vi "InterpolateData.vi"(7 "Interp. factor":i32=4, 8 "error in (no error)":errorcluster, 10 "Time":dbl[](array[numeric]), 11 "Array":cdb[][](array[numeric])) -> (0 "error out":errorcluster, 3 "Array interpolated":cdb[][](array[numeric]))   [LabVIEW 2017, in "AppPlugins.lvlib" / "ModelValidationPlugin.lvclass"]
uses:
  ModelValidationPlugin.lvclass
  <vilib>/gmath/NI_Gmath.lvlib
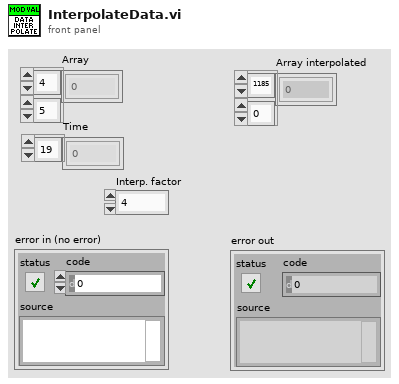
[diagram p1: front panel]
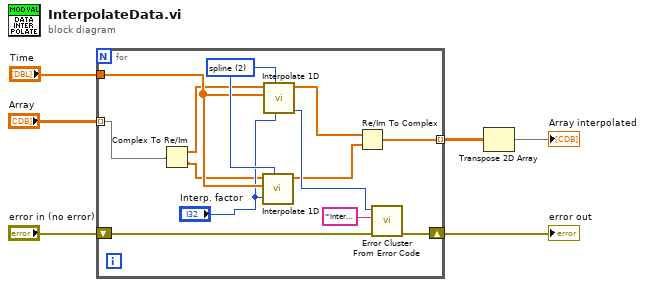
[diagram p0: block diagram]
diagram:
  n1 = for {
    shift-right: [w15] -> w5
    shift-left: "error in (no error)" -> [w16]
    tunnel: "Array" -> [w12] mode=indexing
    tunnel: "Time" -> [w18]
    tunnel: [w7] -> w3 mode=indexing
    w19 = 2 items=["nearest", "linear", "spline", "cubic Hermite", "Lagrange"] ("method")
    n2 = Complex To Re/Im(x + iy=w12) -> (x=w11:dbl[], y=w10:dbl[])
    n3 = call <vilib>:"Interpolate 1D.vi"("ntimes"="Interp. factor", "method"=w19, "X"=w18, "Y"=w10) -> ("yi"=w8:dbl[])  [unwired: 5 in, 2 out]
    n4 = call <vilib>:"Interpolate 1D.vi"("ntimes"="Interp. factor", "method"=w19, "X"=w18, "Y"=w11) -> ("error"=w17:i32, "yi"=w9:dbl[])  [unwired: 5 in, 1 out]
    n5 = Re/Im To Complex(1:w8, 2:w9) -> (0:w7:cdb[])
    n6 = call <vilib>:"Error Cluster From Error Code.vi"("error in (no error)"=w16, "error message (\"\")"="'Interpolatation error: check the interpolation input and parameters'" ("error message (\"\")"), "error code (0)"=w17) -> ("error out"=w15:errorcluster)  [unwired: 6 in]
  }
  "error out" <- w5
  n7 = Transpose 2D Array(2D array=w3) -> (transposed array=→"Array interpolated":cdb[][])
